vi "Part 2.vi"(11 "Input":string) -> (3 "Output":i64)   [LabVIEW 2021]
uses:
  <userlib>/_OpenG.lib/string/string.llb/Convert EOLs (String)__ogtk.vi
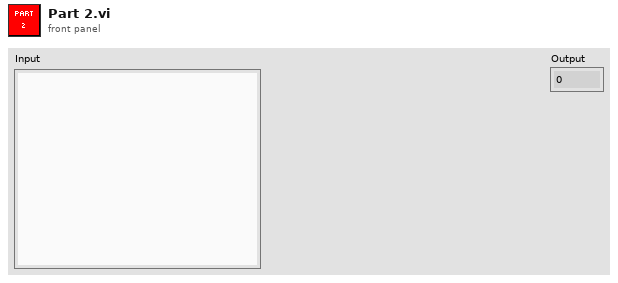
[diagram p1: front panel]
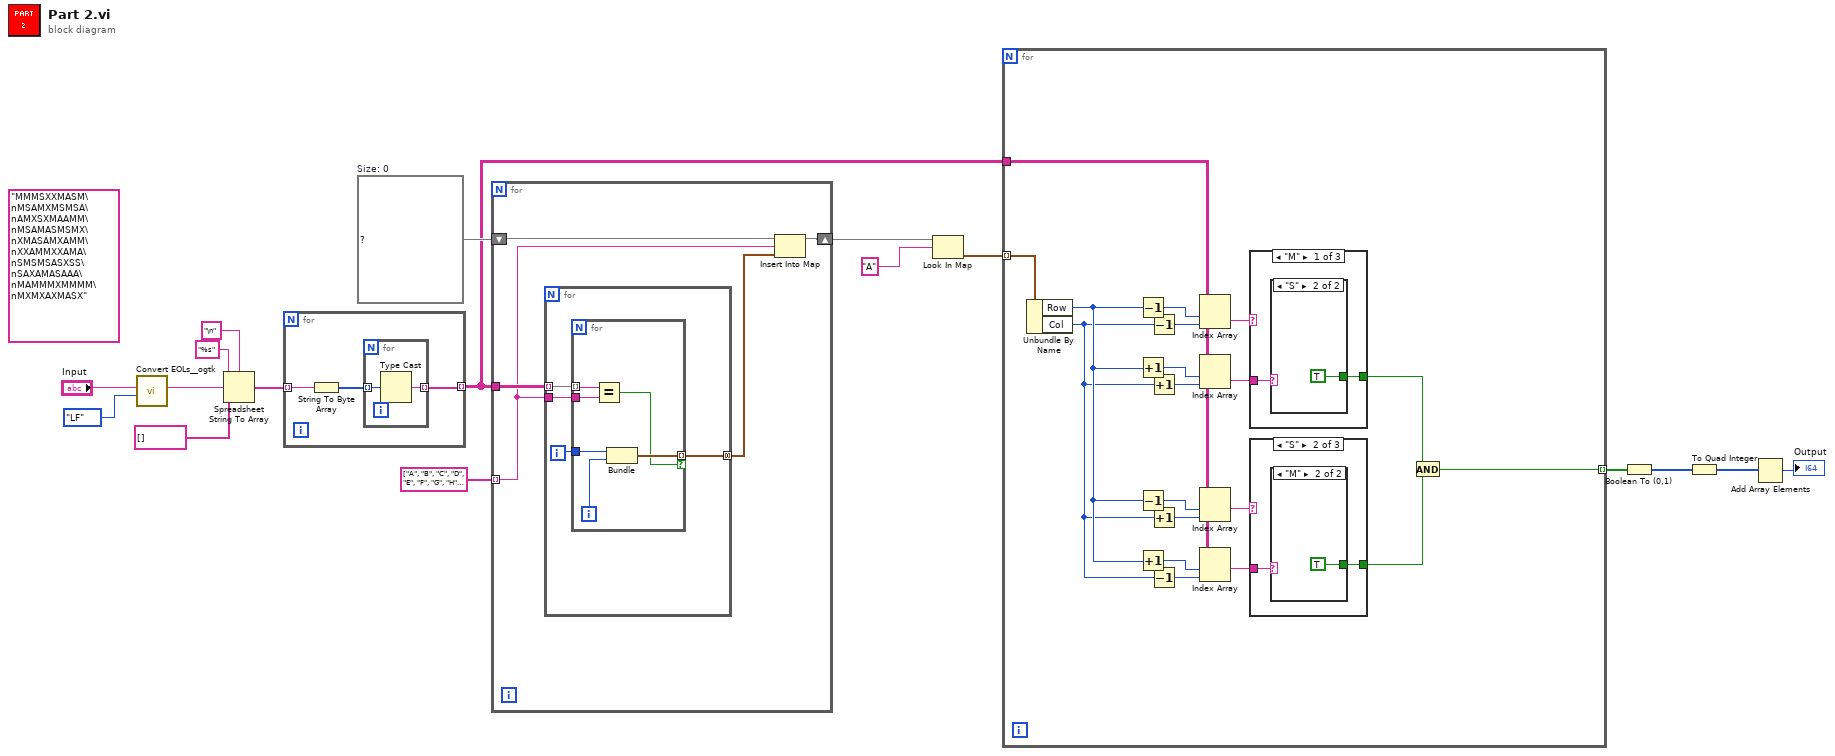
[diagram p0: block diagram]
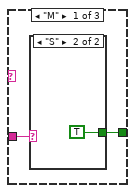
[diagram p2: hidden frame]
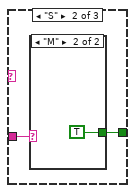
[diagram p7: hidden frame]
diagram:
  (unwired) "MMMSXXMASM\nMSAMXMSMSA\nAMXSXMAAMM\nMSAMASMSMX\nXMASAMXAMM\nXXAMMXXAMA\nSMSMSASXSS\nSAXAMASAAA\nMAMMMXMMMM\nMXMXAXMASX"
  w11 = map{string, cluster{"Row":i32, "Col":i32}[]} {}  # Size: 0
  n1 = call-poly <userlib>:"Convert EOLs__ogtk.vi"("Convert to:"=enum16{"CR", "LF", "CRLF"}."LF", "String in"="Input") -> ("String out"=w14:string)  [unwired: 9 in]
  n2 = Spreadsheet String To Array(delimiter (Tab)="\n", format string="%s", spreadsheet string=w14, array type (2D Dbl)=string[] []) -> (array=w12:string[])
  n3 = for {
    tunnel: w12 -> [w20] mode=indexing
    tunnel: [w18] -> w6 mode=indexing
    n4 = String To Byte Array(string=w20) -> (unsigned byte array=w19:u8[])
    n5 = for {
      tunnel: w19 -> [w22] mode=indexing
      tunnel: [w21] -> w18 mode=indexing
      n6 = Type Cast(x=w22) -> (*(type *) &x=w21:string)  [unwired: 1 in]
    }
  }
  n7 = for {
    tunnel: w6 -> [w25]
    tunnel: string[] ["A", "B", "C", "D", "E", "F", "G", "H", "I", "J", "K", "L", "M", "N", "O", "P", "Q", "R", "S", "T", "U", "V", "W", "X", "Y", "Z"] ("Array") -> [w24] mode=indexing
    shift-right: [w27] -> w10
    shift-left: w11 -> [w26]
    n8 = for {
      tunnel: w25 -> [w31] mode=indexing
      tunnel: w24 -> [w30]
      tunnel: [w28] -> w23 mode=concatenating
      i -> [w29]
      n9 = for {
        tunnel: w31 -> [w37] mode=indexing
        tunnel: w30 -> [w36]
        tunnel: w29 -> [w35]
        tunnel: [w33] -> w28 mode=indexing if=w32
        i -> [w34]
        n10 = Equal?(x=w37, y=w36) -> (x = y?=w32:bool)
        n11 = Bundle(w35, w34) -> (w33:cluster{i32, i32})  [unwired: 1 in]
      }
    }
    n12 = Insert Into Map(map in=w26, key=w24, value=w23) -> (map out=w27:map{string, cluster{"Row":i32, "Col":i32}[]})  [unwired: 2 out]
  }
  n13 = Look In Map(map=w10, key="A") -> (value=w8:cluster{"Row":i32, "Col":i32}[])  [unwired: 1 in, 1 out]
  n14 = for {
    tunnel: w8 -> [w44] mode=indexing
    tunnel: w6 -> [w47]
    tunnel: [w39] -> w5 mode=indexing
    n15 = Unbundle By Name(w44) -> ("Row"=w48:i32, "Col"=w38:i32)
    n16 = Decrement(x=w48) -> (x-1=w56:i32)
    n17 = Increment(x=w48) -> (x+1=w53:i32)
    n18 = Decrement(x=w48) -> (x-1=w49:i32)
    n19 = Increment(x=w48) -> (x+1=w52:i32)
    n20 = Decrement(x=w38) -> (x-1=w55:i32)
    n21 = Increment(x=w38) -> (x+1=w54:i32)
    n22 = Increment(x=w38) -> (x+1=w50:i32)
    n23 = Decrement(x=w38) -> (x-1=w51:i32)
    n24 = Index Array(array=w47, index (row)=w56, index (col)=w55) -> (element=w43:string)
    n25 = Index Array(array=w47, index (row)=w53, index (col)=w54) -> (element=w42:string)
    n26 = Index Array(array=w47, index (row)=w49, index (col)=w50) -> (element=w41:string)
    n27 = Index Array(array=w47, index (row)=w52, index (col)=w51) -> (element=w40:string)
    n28 = case shown="\"M\"" w43 {
      tunnel: w42 -> [w64 w67 _]
      tunnel: [w63 w66 _] -> w46
      frame "M" {
        n29 = case shown="\"S\"" w64 {
          tunnel: [_ TRUE] -> w63
          frame Default {
          }
          frame "S" {
          }
        }
      }
      frame "S" {
        n30 = case shown="\"M\"" w67 {
          tunnel: [_ TRUE] -> w66
          frame Default {
          }
          frame "M" {
          }
        }
      }
      frame Default {
      }
    }
    n31 = case shown="\"S\"" w41 {
      tunnel: w40 -> [w58 w61 _]
      tunnel: [w57 w60 _] -> w45
      frame "M" {
        n32 = case shown="\"S\"" w58 {
          tunnel: [_ TRUE] -> w57
          frame Default {
          }
          frame "S" {
          }
        }
      }
      frame "S" {
        n33 = case shown="\"M\"" w61 {
          tunnel: [_ TRUE] -> w60
          frame Default {
          }
          frame "M" {
          }
        }
      }
      frame Default {
      }
    }
    n34 = And(x=w46, y=w45) -> (x .and. y?=w39:bool)
  }
  n35 = Boolean To (0,1)(Boolean=w5) -> (0, 1=w4:i16[])
  n36 = To Quad Integer(1:w4) -> (0:w2:i64[])
  n37 = Add Array Elements(numeric array=w2) -> (sum=→"Output":i64)
